vi "SF2 Orientation History AE.vi"(7 "Update":bool, 11 "SF2 Buffer (in)":dbl[][](array[numeric]) format="%#_6f") -> (3 "SF2 Buffer (out)":dbl[][](array[numeric]) format="%.10f")   [LabVIEW 2016]
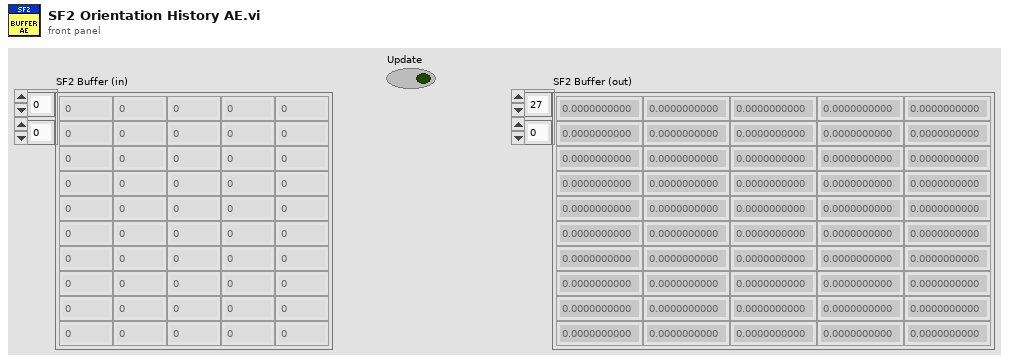
[diagram p1: front panel]
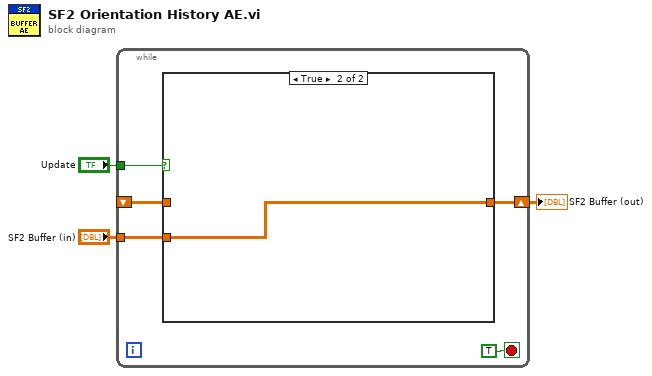
[diagram p0: block diagram]
diagram:
  n1 = while {
    shift-right: [w6] -> w1
    shift-left: _ -> [w4]
    tunnel: "Update" -> [w7]
    tunnel: "SF2 Buffer (in)" -> [w5]
    stop <- TRUE stop-if-true
    n2 = case shown="True" w7 {
      tunnel: [w9 w10] -> w6
      tunnel: w5 -> [_ w10]
      tunnel: w4 -> [w9 _]
      frame False {
      }
      frame True {
      }
    }
  }
  "SF2 Buffer (out)" <- w1
